vi "SCPI_enum_to_string.vi"(1 "SCPI":T1 items=["*IDN?", "*SAV 1", "*RCL 1", "INSTTrument CH1", "INSTTrument CH2", "INSTrument?", "MEASure:CURRent? CH1", "MEASure:CURRent? CH2", "MEASure:VOLTage? CH1", "MEASure:VOLTage? CH2", "MEASure:POWEr? CH1", "MEASure:POWEr? CH2", "CH1:CURRent?", "CH2:CURRent?", "CH1:VOLTage? ", "CH2:VOLTage? ", "OUTPut CH1,ON", "OUTPut CH1,OFF", "OUTPut CH2,ON", "OUTPut CH2,OFF", "OUTPut CH3,ON", "OUTPut CH3,OFF", "OUTPut:TRACK 0", "OUTPut:TRACK 1", "OUTPut:TRACK 2", "OUTPut:WAVE CH1,ON", "OUTPut:WAVE CH1,OFF", "OUTPut:WAVE CH2,ON", "OUTPut:WAVE CH2,OFF", "CH1:VOLTage ", "CH2:VOLTage ", "CH1:CURRent ", "CH2:CURRent "]) -> (0 "resulting string 2":string)   [LabVIEW 2020]
doc: "enum (ONLY SCPI TYP DEF) to string\n\nconvert chosen index of enum to string"
uses:
  controls/SCPI_enum.ctl
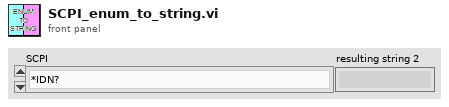
[diagram p1: front panel]
types:
  T1 = typedef "SCPI_enum.ctl" = u16
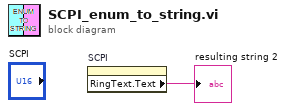
[diagram p0: block diagram]
diagram:
  n1 = property on="SCPI" class="Ring (strict)"() -> ("RingText.Text"=→"resulting string 2":string)  [unwired: 2 in, 2 out]
